vi "FT10_Connect Hardware.vi"(0 "Message Handling Cluster in":T1={"Fornax Connected?"=refnum, "Unitherm Connected?"=refnum, "M4X Connected?"=refnum, "Unitherm Connect/Disconnect"=refnum, "Fornax Connection"=refnum, "UNITHERM Connection"="", "M4X Connection"=0, "PXI-7854R FPGA Reference"=refnum, "PXI-7854R Connected?"=refnum, "Fornax Connect/Disconnect"=refnum, "7854 Connect/Disconnect"=refnum, "M4X Connect/Disconnect"=refnum, "Config Cluster"={"Unitherm Port"="COM4", "Simulate Values"=TRUE}, "Log Queue"=refnum, "Log Analysis Cluster"={"RMS"=0.0, "Envelope Frequency"=0.0, "Peak"=0.0, "Crest Factor"=0.0, "Duty Cyle %"=0.0, "P-P"=0.0, "Frequency"=0.0, "THD"=0.0, "Postive Peak"=0.0, "Negative Peak"=0.0, "Mag_H1"=0.0, "Phase_H1"=0.0, "Mag_H3"=0.0, "Phase_H3"=0.0, "Mag_H5"=0.0, "Phase_H5"=0.0}, "Log Waveform Cluster"={"t0"=timestamp(0 s since 1904-01-01), "dt"=1.0, "Y"=[]}, "Log Time"=timestamp(0 s since 1904-01-01), "Log Flag"=FALSE}, 11 "error in (no error)":errorcluster) -> (4 "Message Handling Cluster out":T1={"Fornax Connected?"=refnum, "Unitherm Connected?"=refnum, "M4X Connected?"=refnum, "Unitherm Connect/Disconnect"=refnum, "Fornax Connection"=refnum, "UNITHERM Connection"="", "M4X Connection"=0, "PXI-7854R FPGA Reference"=refnum, "PXI-7854R Connected?"=refnum, "Fornax Connect/Disconnect"=refnum, "7854 Connect/Disconnect"=refnum, "M4X Connect/Disconnect"=refnum, "Config Cluster"={"Unitherm Port"="COM4", "Simulate Values"=TRUE}, "Log Queue"=refnum, "Log Analysis Cluster"={"RMS"=0.0, "Envelope Frequency"=0.0, "Peak"=0.0, "Crest Factor"=0.0, "Duty Cyle %"=0.0, "P-P"=0.0, "Frequency"=0.0, "THD"=0.0, "Postive Peak"=0.0, "Negative Peak"=0.0, "Mag_H1"=0.0, "Phase_H1"=0.0, "Mag_H3"=0.0, "Phase_H3"=0.0, "Mag_H5"=0.0, "Phase_H5"=0.0}, "Log Waveform Cluster"={"t0"=timestamp(0 s since 1904-01-01), "dt"=1.0, "Y"=[]}, "Log Time"=timestamp(0 s since 1904-01-01), "Log Flag"=FALSE}, 6 "Fornax Connected?":bool, 8 "Unitherm Connected?":bool, 10 "M4X Connected?":bool, 14 "PXI-7854R Connected?":bool, 15 "error out":errorcluster)   [LabVIEW 2015]
doc: "Connects to Fornax, Unitherm, PXIe, and M4X. Then bundles connections into cluster."
uses:
  Controls/Control_Message Handling Cluster.ctl
  Controls/Control_M4X Connection.ctl
  Controls/Control_PXI-7854R FPGA Reference.ctl
  Controls/Control_Config Cluster.ctl
  Controls/Control_Config Unitherm Port.ctl
  Controls/Control_Config Simulate Values.ctl
  Controls/Control_Log Queue.ctl
  Controls/Control_Log Cluster.ctl
  Controls/Control_Log Time.ctl
  Controls/Control_Log Waveform Cluster.ctl
  Controls/Control_Log Analysis Cluster.ctl
  Controls/Control_Log Flag.ctl
  <vilib>/userdefined/High Color/nirio_resource_hc.ctl
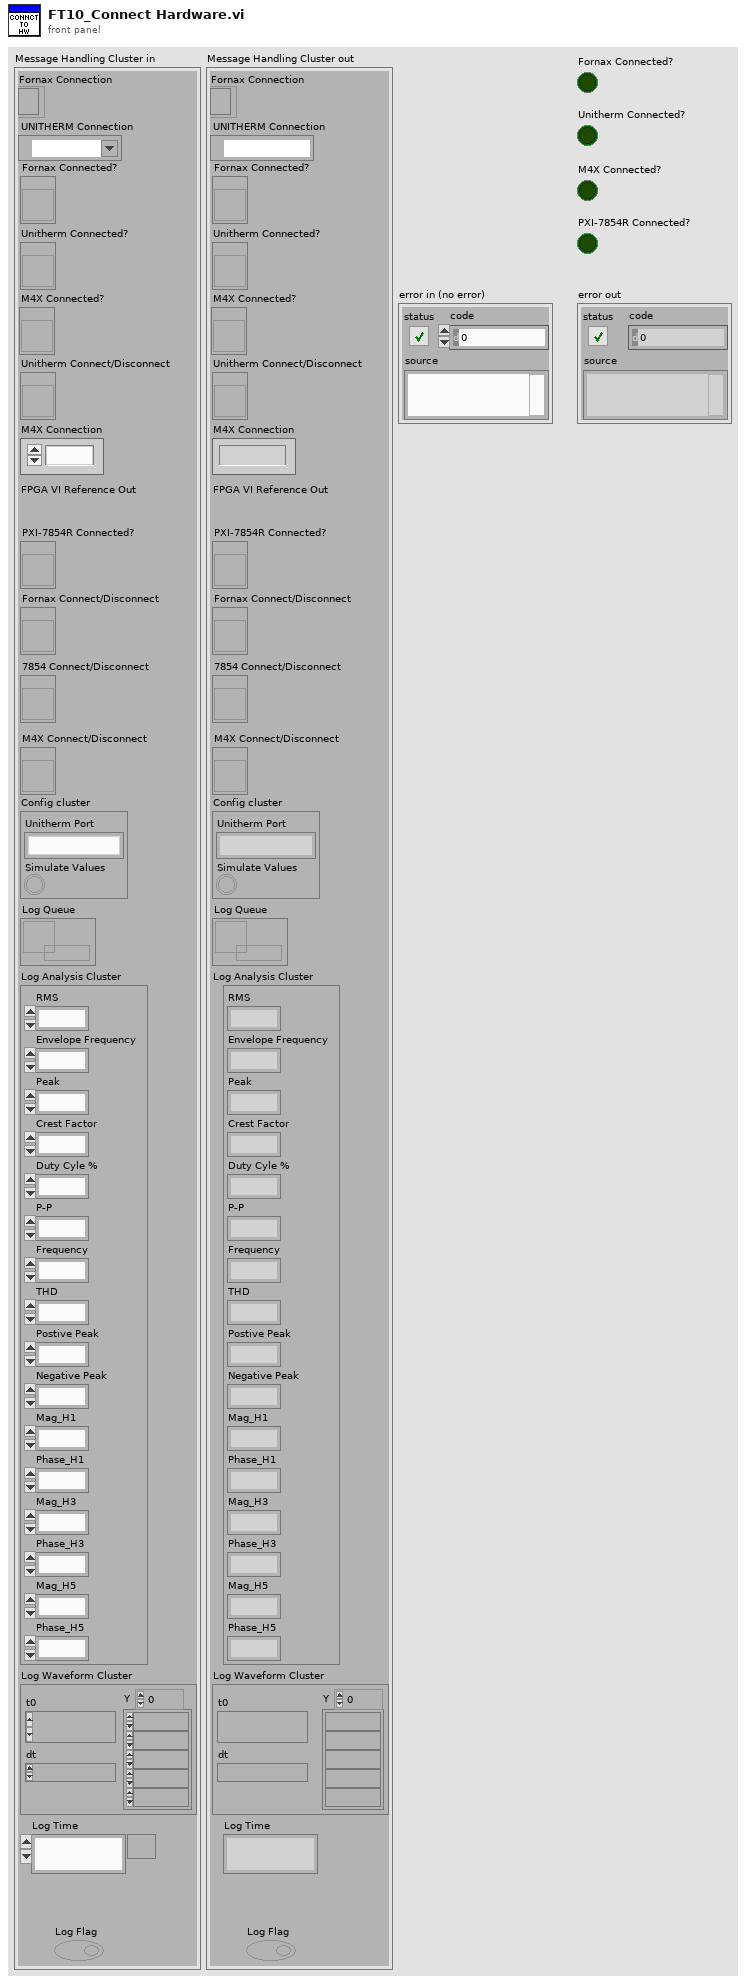
[diagram p1: front panel]
types:
  T1 = typedef "Control_Message Handling Cluster.ctl" = cluster{"Fornax Connected?":refnum<vi>, "Unitherm Connected?":refnum<vi>, "M4X Connected?":refnum<vi>, "Unitherm Connect/Disconnect":refnum<vi>, "Fornax Connection":refnum<k5>, "UNITHERM Connection":refnum<visa-resource-name>, "M4X Connection":T2, "PXI-7854R FPGA Reference":T3, "PXI-7854R Connected?":refnum<vi>, "Fornax Connect/Disconnect":refnum<vi>, "7854 Connect/Disconnect":refnum<vi>, "M4X Connect/Disconnect":refnum<vi>, "Config Cluster":T4, "Log Queue":T7, "Log Analysis Cluster":T8, "Log Waveform Cluster":T9, "Log Time":T10, "Log Flag":T11}
  T2 = typedef "Control_M4X Connection.ctl" = u32
  T3 = typedef "Control_PXI-7854R FPGA Reference.ctl" = refnum<k20>
  T4 = typedef "Control_Config Cluster.ctl" = cluster{"Unitherm Port":T5, "Simulate Values":T6}
  T5 = typedef "Control_Config Unitherm Port.ctl" = string
  T6 = typedef "Control_Config Simulate Values.ctl" = bool
  T7 = typedef "Control_Log Queue.ctl" = refnum<queue>
  T8 = typedef "Control_Log Analysis Cluster.ctl" = cluster{"RMS":dbl, "Envelope Frequency":dbl, "Peak":dbl, "Crest Factor":dbl, "Duty Cyle %":dbl, "P-P":dbl, "Frequency":dbl, "THD":dbl, "Postive Peak":dbl, "Negative Peak":dbl, "Mag_H1":dbl, "Phase_H1":dbl, "Mag_H3":dbl, "Phase_H3":dbl, "Mag_H5":dbl, "Phase_H5":dbl}
  T9 = typedef "Control_Log Waveform Cluster.ctl" = waveform(dbl)
  T10 = typedef "Control_Log Time.ctl" = timestamp
  T11 = typedef "Control_Log Flag.ctl" = bool
  T12 = typedef "nirio_resource_hc.ctl" = tag
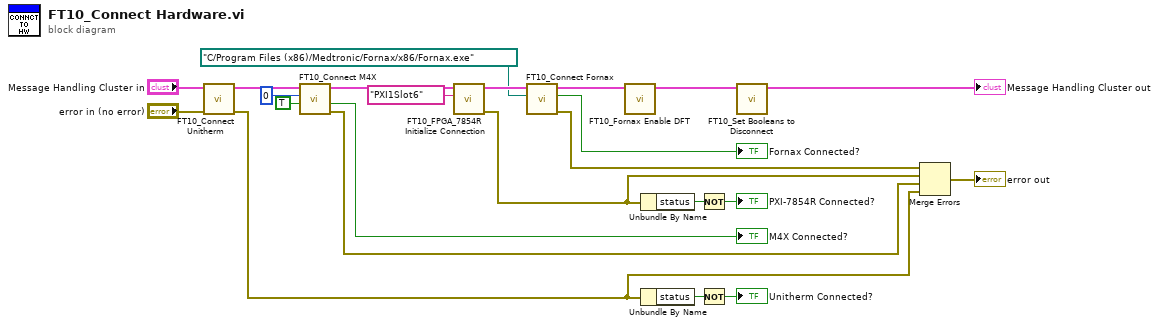
[diagram p0: block diagram]
diagram:
  n1 = call "FT10_Connect Unitherm.vi"("error in (no error)"="error in (no error)", "Message Handling Cluster in"="Message Handling Cluster in") -> ("error out"=w6:errorcluster, "Message Handling Cluster out"=w5:T1)  [unwired: 8 in]
  n2 = call "FT10_Connect M4X.vi"("reset device"=TRUE, "Board #"=u32 0, "Message Handling Cluster in"=w5) -> ("error out"=w13:errorcluster, "M4X Connected?"=→"M4X Connected?":bool, "Message Handling Cluster out"=w14:T1)  [unwired: 5 in, 1 out]
  n3 = call "FT10_FPGA_7854R Initialize Connection.vi"("FPGA resource name"=T12 "PXI1Slot6", "Message Handling Cluster in"=w14) -> ("error out"=w12:errorcluster, "Message Handling Cluster out"=w9:T1)  [unwired: 7 in, 1 out]
  n4 = call "FT10_Connect Fornax.vi"("Fornax Executable Path"=path "C:/Program Files (x86)/Medtronic/Fornax/x86/Fornax.exe", "Message Handling Cluster in"=w9) -> ("error out"=w21:errorcluster, "Fornax Connected?"=→"Fornax Connected?":bool, "Message Handling Cluster out"=w3:T1)  [unwired: 7 in]
  n5 = call "FT10_Fornax Enable DFT.vi"("Message Handling Cluster in"=w3) -> ("Message Handling Cluster out"=w2:T1)  [unwired: 10 in]
  n6 = Unbundle By Name(w12) -> ("status"=w11:bool)
  n7 = Unbundle By Name(w6) -> ("status"=w22:bool)
  n8 = Not(x=w11) -> (.not. x?=→"PXI-7854R Connected?":bool)
  n9 = Not(x=w22) -> (.not. x?=→"Unitherm Connected?":bool)
  n10 = call "FT10_Set Booleans to Disconnect.vi"("Message Handling Cluster in"=w2) -> ("Message Handling Cluster out"=→"Message Handling Cluster out":T1)  [unwired: 10 in]
  n11 = Merge Errors(w21, w12, w13, w6) -> (→"error out":errorcluster)
